vi "nominal.is_token_valid.vi"(8 "error in (no error)":errorcluster, 11 "token":path) -> (0 "error out":errorcluster, 3 "valid":bool)   [LabVIEW 2024]
uses:
  <vilib>/Nominal/Nominal IO Client/Nominal Client/Nominal Client.lvclass/Nominal Client.ctl
  c13ba591-26ac-4ac6-a0cd-7939f5a04ff7.vi
  <vilib>/Nominal/Nominal IO Client/Nominal Client/private_data.set.vi
  <vilib>/Utility/error.llb/Error Cluster From Error Code.vi
  <vilib>/addons/_JKI.lib/REST Client/classes/REST Client/Create REST Client.vi
  <vilib>/Nominal/Nominal IO Client/Nominal Client/Nominal Client.lvclass
  <vilib>/addons/_JKI.lib/REST Client/classes/REST Client/REST Client.lvclass
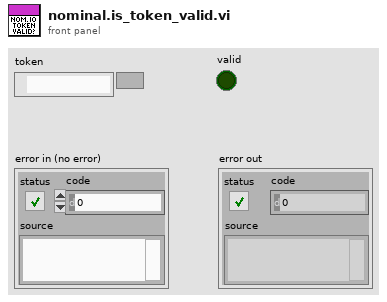
[diagram p1: front panel]
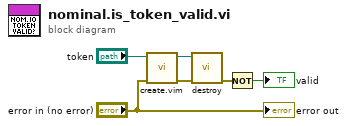
[diagram p0: block diagram]
diagram:
  n1 = call "create.vim"("error in"="error in (no error)", "API Token (string or path)"="token") -> ("error out"=w5:errorcluster, "Nominal Client"=w6:refnum<class "Nominal Client.lvclass">)  [unwired: 8 in]
  n2 = call <vilib>:"destroy.vi"("error in"=w5, "Nominal Client"=w6) -> ("error out"=w3:errorcluster)  [unwired: 9 in]
  n3 = Not(x=w3) -> (.not. x?=→"valid":bool)
  "error out" <- "error in (no error)"
